vi "Write Message Forward Target Type.vi"(8 "error in (no error)":errorcluster, 10 "Message Forward Target Type":T1 caption="Enum 3", 11 "Node Actor MSG in":refnum<class "Node Actor MSG.lvclass">) -> (0 "error out":errorcluster, 3 "Node Actor MSG out":refnum<class "Node Actor MSG.lvclass">)   [LabVIEW 2024, in "Node Actor MSG.lvclass"]
uses:
  Node Actor MSG.lvclass
  Node Actor MSG.lvclass/Node Actor MSG.ctl
  Type Def/Message Forward Target Type.ctl
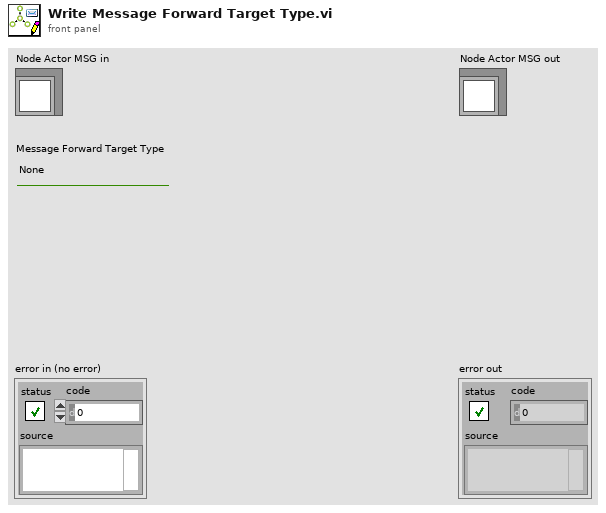
[diagram p1: front panel]
types:
  T1 = typedef "Message Forward Target Type.ctl" = enum16{"None", "ID", "Tag", "Mail Startegy", "Task"}
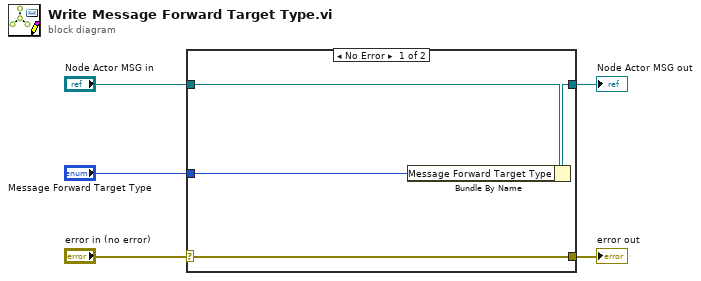
[diagram p0: block diagram]
diagram:
  n1 = case shown="No Error" "error in (no error)" {
    selector: "error in (no error)" -> [w9 w10]
    tunnel: [w9 w10] -> w4
    tunnel: [w7 w11] -> w2
    tunnel: "Node Actor MSG in" -> [w8 w11]
    tunnel: "Message Forward Target Type" -> [w6 _]
    frame No Error {
      n2 = Bundle By Name(cluster=w8, "Message Forward Target Type"=w6) -> (w7:refnum<class "Node Actor MSG.lvclass">)
    }
    frame Error {
    }
  }
  "error out" <- w4
  "Node Actor MSG out" <- w2
